vi "App.Save.vi"(8 "error in (no error)":errorcluster, 10 "selected path":path, 11 "State Variables":T1={"Aliases.All"=[], "Aliases.Outputs"=[], "UI.Sequence#ofColumns"=0, "SysDef.Path"=path "", "UI.SequenceRef"=refnum, "UI.StepInformationRef"=refnum, "UI.AbortRef"=refnum, "UI.GraphRef"=refnum, "UI.ViewRef"=refnum, "UI.IterationsRef"=refnum, "UI.IterationInformationRef"=refnum, "INI.Settings"={"Build Location"=path "C:/Simple Sequence Editor/SequenceRepo", "LoggingLocation"=path ""}, "NIVS.Workspace Event"=refnum, "UI.SkipChannel"=refnum, "NIVS.Launched?"=FALSE}) -> (0 "error out":errorcluster)   [LabVIEW 2013, in "Simple Sequence Tools - Editor.lvlib"]
uses:
  Simple Sequence Tools - Editor.lvlib
  Types/Main.StateVariables.ctl
  Shared/Types/Channel.Properties.ctl
  Shared/Types/INI.Settings
  Shared/Types/Saved.Sequence.ctl
  Shared/Simple Sequence Tools - Shared.lvlib
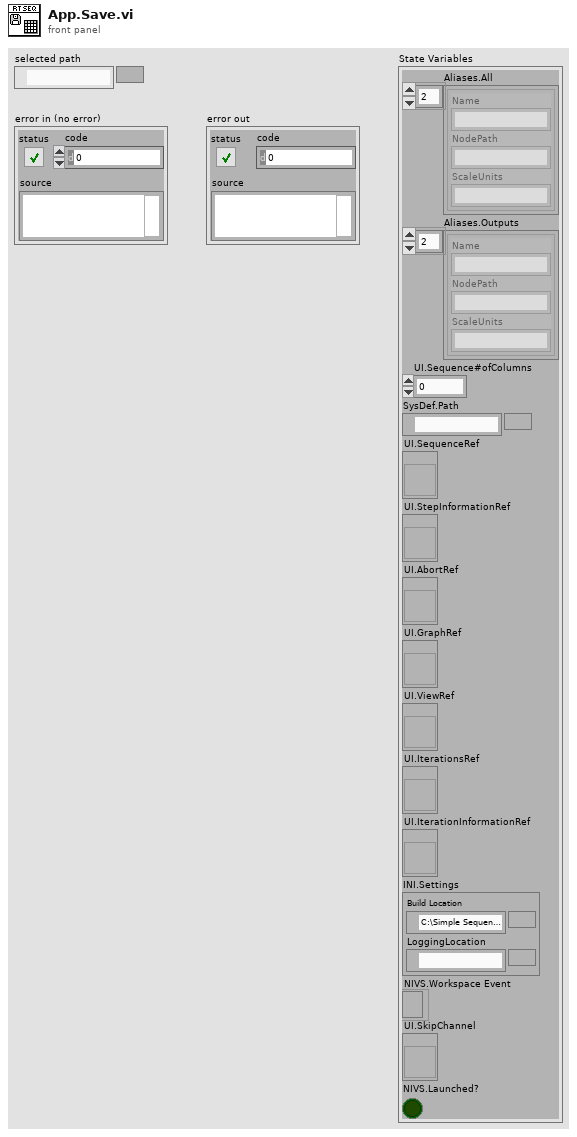
[diagram p1: front panel]
types:
  T1 = typedef "Simple Sequence Tools - Editor.lvlib/Main.StateVariables.ctl" = cluster{"Aliases.All":T2[], "Aliases.Outputs":T2[], "UI.Sequence#ofColumns":i32, "SysDef.Path":path, "UI.SequenceRef":refnum<vi>, "UI.StepInformationRef":refnum<vi>, "UI.AbortRef":refnum<vi>, "UI.GraphRef":refnum<vi>, "UI.ViewRef":refnum<vi>, "UI.IterationsRef":refnum<vi>, "UI.IterationInformationRef":refnum<vi>, "INI.Settings":T3, "NIVS.Workspace Event":refnum<event-registration>, "UI.SkipChannel":refnum<vi>, "NIVS.Launched?":bool}
  T2 = typedef "Simple Sequence Tools - Shared.lvlib/Channel.Properties.ctl" = cluster{"Name":string, "NodePath":string, "ScaleUnits":string}
  T3 = typedef "Simple Sequence Tools - Shared.lvlib/INI.Settings" = cluster{"Build Location":path, "LoggingLocation":path}
  T4 = typedef "Simple Sequence Tools - Shared.lvlib/Saved.Sequence.ctl" = cluster{"Output Channels":T2[], "Item Names":string[][], "Step":string, "Abort":string, "Iterations":u32, "Iteration":string, "Skip":string}
  T5 = enum16{"open", "replace", "create", "open or create", "replace or create", "replace or create with confirmation"}
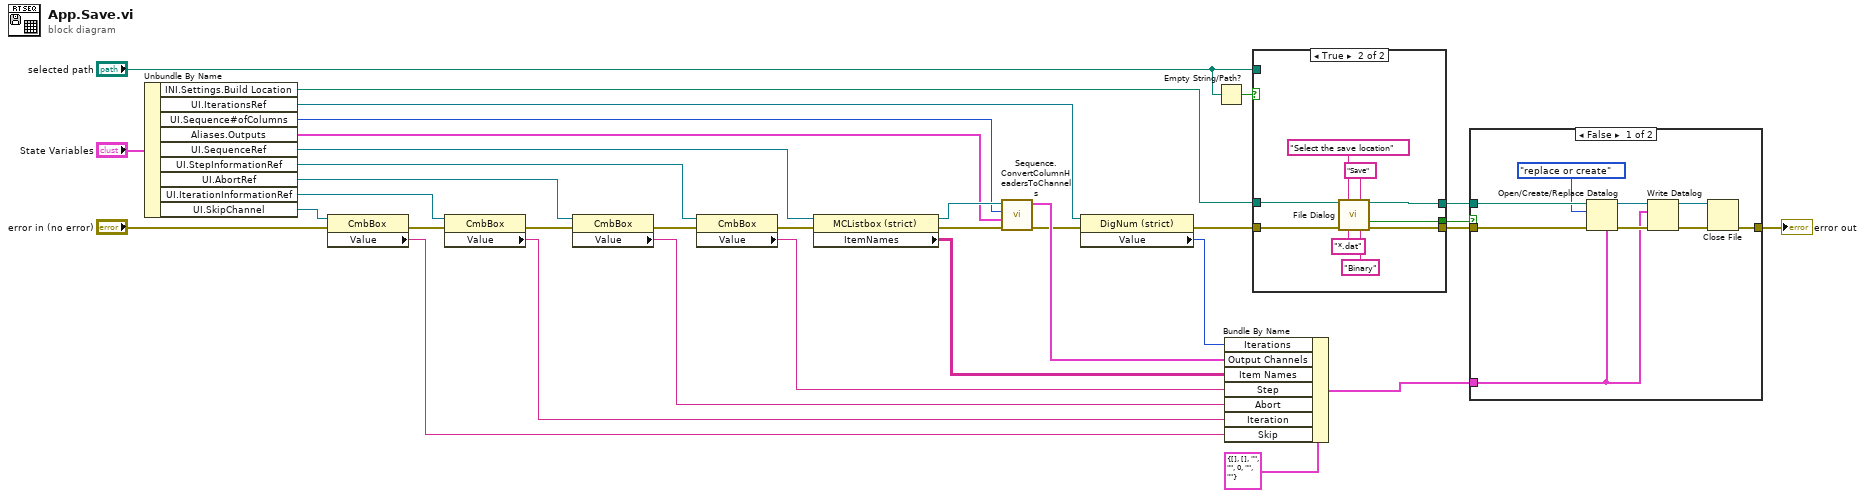
[diagram p0: block diagram]
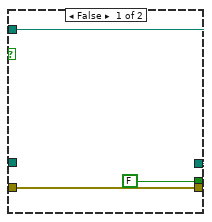
[diagram p2: hidden frame]
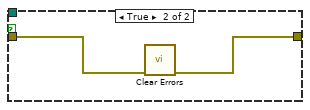
[diagram p3: hidden frame]
diagram:
  n1 = Unbundle By Name("State Variables") -> ("INI.Settings.Build Location"=w5:path, "UI.IterationsRef"=w19:refnum<vi>, "UI.Sequence#ofColumns"=w12:i32, "Aliases.Outputs"=w11:T2[], "UI.SequenceRef"=w20:refnum<vi>, "UI.StepInformationRef"=w26:refnum<vi>, "UI.AbortRef"=w27:refnum<vi>, "UI.IterationInformationRef"=w18:refnum<vi>, "UI.SkipChannel"=w4:refnum<vi>)
  n2 = property class="CmbBox"(reference=w4, error in="error in (no error)") -> (error out=w2:errorcluster, "Value"=w1:string)  [unwired: 1 out]
  n3 = property class="CmbBox"(reference=w18, error in=w2) -> (error out=w17:errorcluster, "Value"=w9:string)  [unwired: 1 out]
  n4 = property class="CmbBox"(reference=w27, error in=w17) -> (error out=w28:errorcluster, "Value"=w33:string)  [unwired: 1 out]
  n5 = property class="CmbBox"(reference=w26, error in=w28) -> (error out=w29:errorcluster, "Value"=w32:string)  [unwired: 1 out]
  n6 = property class="MCListbox (strict)"(reference=w20, error in=w29) -> (reference out=w13:refnum<vi>, error out=w16:errorcluster, "ItemNames"=w8:string[][])
  n7 = call "Sequence.ConvertColumnHeadersToChannels.vi"("error in (no error)"=w16, "Aliases.Outputs"=w11, "UI.Sequence#ofColumns"=w12, "UI.SequenceRef"=w13) -> ("error out"=w15:errorcluster, "Output Channels"=w31:T2[])  [unwired: 5 in, 1 out]
  n8 = property class="DigNum (strict)"(reference=w19, error in=w15) -> (error out=w14:errorcluster, "Value"=w10:u32)  [unwired: 1 out]
  n9 = Empty String/Path?(string/path="selected path") -> (empty?=w7:bool)
  n10 = Bundle By Name(cluster=T4 {"Output Channels"=[], "Item Names"=[], "Step"="", "Abort"="", "Iterations"=0, "Iteration"="", "Skip"=""}, "Iterations"=w10, "Output Channels"=w31, "Item Names"=w8, "Step"=w32, "Abort"=w33, "Iteration"=w9, "Skip"=w1) -> (w34:T4)
  n11 = case shown="True" w7 {
    tunnel: [FALSE ("cancelled") w45] -> w24
    tunnel: [w35 w44] -> w23
    tunnel: [w37 w40] -> w22
    tunnel: w14 -> [w37 w38]
    tunnel: "selected path" -> [w35 _]
    tunnel: w5 -> [_ w39]
    frame False {
    }
    frame True {
      n12 = call "File Dialog"("start path"=w39, "prompt"="Select the save location", "button label"="Save", "error in"=w38, "pattern (all files)"="*.dat", "pattern label"="Binary") -> ("selected path"=w44:path, "cancelled"=w45:bool, "error out"=w40:errorcluster)  [unwired: 6 in, 1 out]
    }
  }
  n13 = case shown="False" w24 {
    tunnel: [w55 w56] -> w21
    tunnel: w22 -> [w52 w57]
    tunnel: w23 -> [w54 _]
    tunnel: w34 -> [w48 _]
    frame False {
      n14 = Open/Create/Replace Datalog(5:w48, 8:w52, 10:T5."replace or create" ("operation (0:open)"), 11:w54) -> (0:w51:errorcluster, 3:w49:refnum<k1>)  [unwired: 2 in, 1 out]
      n15 = Write Datalog(4:w51, 6:w48, 7:w49) -> (0:w50:errorcluster, 3:w47:refnum<k1>)
      n16 = Close File(refnum=w47, error in=w50) -> (error out=w55:errorcluster)  [unwired: 1 out]
    }
    frame True {
      n17 = call <vilib>:"Clear Errors.vi"("error in (no error)"=w57) -> ("error out"=w56:errorcluster)  [unwired: 6 in]
    }
  }
  "error out" <- w21
